vi "Table Trim Whites.vi"(8 "error in":errorcluster, 11 "table ref":refnum<vi>) -> (0 "error out":errorcluster, 2 "reduced array":string[][](array[string]), 3 "table ref out":refnum<vi>)   [LabVIEW 2020]
doc: "Reduces size of array to minimum non-white rectangle."
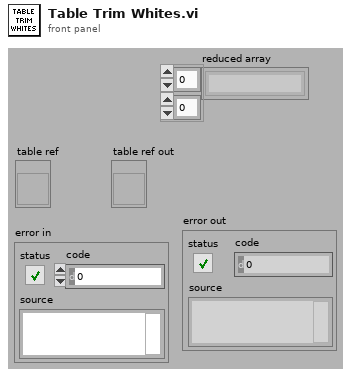
[diagram p1: front panel]
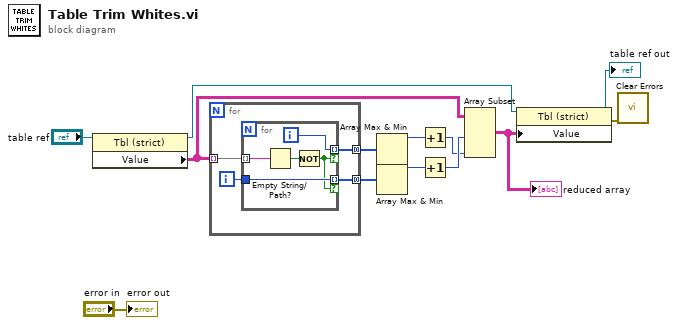
[diagram p0: block diagram]
diagram:
  n1 = property on="Property Node" class="Tbl (strict)"(reference="table ref") -> (reference out=w6:refnum<vi>, "Value"=w8:string[][])  [unwired: 1 in, 1 out]
  n2 = for {
    tunnel: w8 -> [w17] mode=indexing
    tunnel: [w15] -> w12 mode=concatenating
    tunnel: [w14] -> w10 mode=concatenating
    i -> [w16]
    n3 = for {
      tunnel: w17 -> [w22] mode=indexing
      tunnel: [w21] -> w15 mode=indexing if=w18
      tunnel: [w19] -> w14 mode=indexing if=w18
      tunnel: w16 -> [w19]
      i -> [w21]
      n4 = Empty String/Path?(string/path=w22) -> (empty?=w20:bool)
      n5 = Not(x=w20) -> (.not. x?=w18:bool)
    }
  }
  n6 = Array Max & Min(array=w12) -> (max value=w11:i32)  [unwired: 3 out]
  n7 = Array Max & Min(array=w10) -> (max value=w9:i32)  [unwired: 3 out]
  n8 = Increment(x=w11) -> (x+1=w1:i32)
  n9 = Increment(x=w9) -> (x+1=w2:i32)
  n10 = Array Subset(array=w8, length (row)=w2, length (col)=w1) -> (w7:string[][])  [unwired: 2 in]
  "reduced array" <- w7
  n11 = property on="Property Node" class="Tbl (strict)"(reference=w6, "Value"=w7) -> (reference out=→"table ref out":refnum<vi>, error out=w5:errorcluster)  [unwired: 1 in]
  n12 = call <vilib>:"Clear Errors.vi"("error in (no error)"=w5) -> ()  [unwired: 5 in, 2 out]
  "error out" <- "error in"
